vi "Xbox 2nd.vi"() -> (14 "Turn?":bool, 16 "Fire?":bool, 17 "Repelling Balls?":bool, 18 "Right Side?":bool, 19 "Collecting Balls?":bool, 20 "Viewer Select":T2(ring)=enum."Ball Camera", 21 "Hoop Select":T1(ring), 22 "Number Of Balls":i32, 23 "Shooting Manual Override?":bool, 24 "Ball Managment Manual Override?":bool, 25 "No Target Alert":bool, 26 "Manual Override Engaged?":bool, 27 "Aligning?":bool)   [LabVIEW 2011]
uses:
  Team Code/Robot Global Data.vi
panel:
  out "Current RPM":dbl
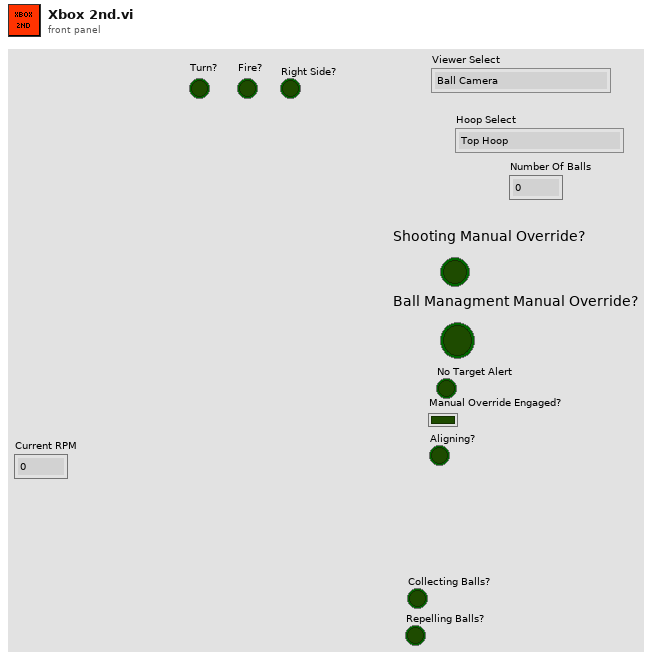
[diagram p1: front panel]
types:
  T1 = enum32{"Top Hoop", "Bottom Hoop", "Left Hoop", "Right Hoop"}
  T2 = enum32{"Target Camera", "Target Camera Mask", "Ball Camera", "Kinect Skeleton"}
  T3 = typedef "WPI_JoystickButtonState.ctl" = cluster{"Button 1":bool, "Button 2":bool, "Button 3":bool, "Button 4":bool, "Button 5":bool, "Button 6":bool, "Button 7":bool, "Button 8":bool, "Button 9":bool, "Button 10":bool, "Button 11":bool, "Button 12":bool}
  T4 = cluster{"Buttons":T3, "Axes":cluster{"axis 1 (x)":dbl, "axis 2 (y)":dbl, "axis 3 (throttle)":dbl, "axis 4":dbl, "axis 5":dbl, "axis 6":dbl}}
  T5 = cluster{"Position":cluster{"X Angle":dbl, "Raw Y":dbl, "Raw X":dbl}, "Distance (ft)":dbl, "BB Angle":dbl}
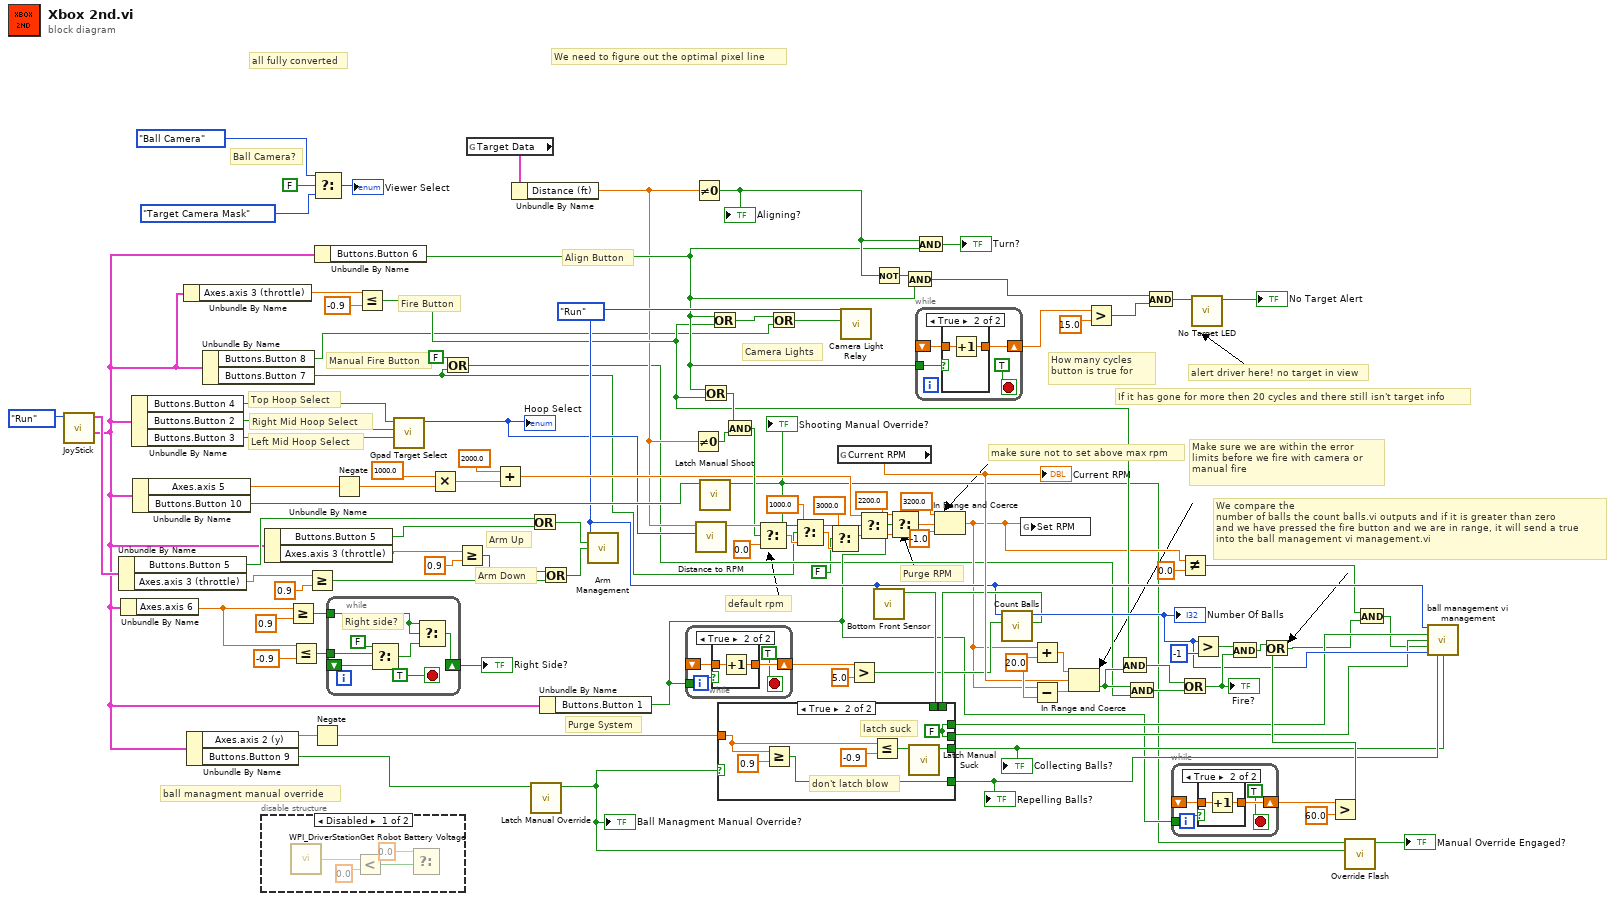
[diagram p0: block diagram]
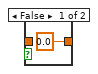
[diagram p2: hidden frame]
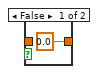
[diagram p4: hidden frame]
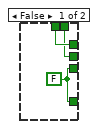
[diagram p5: hidden frame]
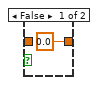
[diagram p6: hidden frame]
diagram:
  w96 = 20.0 ("y")
  w44 = enum16{"Init", "Run", "End"}."Run" ("Enum")
  # "all fully converted"
  # "default rpm"
  # "Make sure we are within the error limits before we fire with camera or manual fire"
  # "make sure not to set above max rpm"
  # "Purge System"
  # "Left Mid Hoop Select"
  # "Right Mid Hoop Select"
  # "Top Hoop Select"
  # "Purge RPM"
  # "We compare the \nnumber of balls the count balls.vi outputs and if it is greater than zero \nand we have pressed the fire button and we are in range, it will send a true\ninto the ball management vi management.vi"
  # "ball managment manual override"
  # "We need to figure out the optimal pixel line"
  # "Arm Down"
  # "Arm Up"
  # "Ball Camera?"
  # "Fire Button"
  # "Manual Fire Button"
  # "Camera Lights"
  # "Align Button"
  # "If it has gone for more then 20 cycles and there still isn't target info"
  # "How many cycles button is true for"
  # "alert driver here! no target in view"
  n1 = call "JoyStick.vi"("Enum"=enum16{"Init", "Run", "End"}."Run") -> ("JoyStick 3"=w34:T4, "JoyStick 1"=w43:T4)  [unwired: 7 in, 2 out]
  n2 = Unbundle By Name(w43) -> ("Buttons.Button 5"=w36:bool, "Axes.axis 3 (throttle)"=w30:dbl)
  n3 = Unbundle By Name(w34) -> ("Axes.axis 6"=w85:dbl)
  n4 = Unbundle By Name(w34) -> ("Buttons.Button 4"=w65:bool, "Buttons.Button 2"=w91:bool, "Buttons.Button 3"=w90:bool)
  n5 = Unbundle By Name(w34) -> ("Axes.axis 5"=w80:dbl, "Buttons.Button 10"=w60:bool)
  n6 = Unbundle By Name(w34) -> ("Axes.axis 3 (throttle)"=w32:dbl)
  n7 = Unbundle By Name(w34) -> ("Axes.axis 2 (y)"=w58:dbl, "Buttons.Button 9"=w59:bool)
  n8 = Unbundle By Name(w34) -> ("Buttons.Button 8"=w1:bool, "Buttons.Button 7"=w6:bool)
  n9 = disable-structure shown="Disabled" {
    frame Disabled {
      n10 = call <vilib>:"WPI_DriverStationGet Robot Battery Voltage.vi"() -> ("robot battery voltage"=w112:dbl)  [unwired: 14 in, 1 out]
      n11 = Less?(x=w112, y=0.0) -> (x < y?=w110:bool)
      n12 = Select(t=0.0, s=w110) -> ()  [unwired: 1 in, 1 out]
    }
    frame Enabled {
    }
  }
  n13 = Unbundle By Name(w34) -> ("Buttons.Button 5"=w37:bool, "Axes.axis 3 (throttle)"=w28:dbl)
  n14 = Greater Or Equal?(x=w85, y=0.9) -> (x >= y?=w83:bool)
  n15 = Less Or Equal?(x=w85, y=-0.9) -> (x <= y?=w82:bool)
  n16 = Greater Or Equal?(x=w30, y=0.9) -> (x >= y?=w29:bool)
  n17 = Negate(x=w58) -> (-x=w66:dbl)
  n18 = Select(t=T2."Ball Camera" ("Viewer Select"), s=FALSE, f=T2."Target Camera Mask" ("Viewer Select")) -> (s? t:f=→"Viewer Select":T2)
  n19 = Unbundle By Name(w34) -> ("Buttons.Button 6"=w40:bool)
  n20 = while {
    tunnel: w83 -> [w115]
    tunnel: w82 -> [w116]
    shift-right: [w117] -> w81
    shift-left: _ -> [w118]
    stop <- TRUE stop-if-true
    # "Right side?"
    n21 = Select(t=FALSE, s=w116, f=w118) -> (s? t:f=w119:bool)
    n22 = Select(t=w115, s=w115, f=w119) -> (s? t:f=w117:bool)
  }
  "Right Side?" <- w81
  n23 = Negate(x=w80) -> (-x=w67:dbl)
  n24 = Less Or Equal?(x=w32, y=-0.9) -> (x <= y?=w31:bool)
  n25 = call "Gpad Target Select.vi"("Left Hoop"=w90, "Right Hoop"=w91, "Top Hoop"=w65) -> ("Hoop Select"=w38:T1)  [unwired: 8 in]
  "Hoop Select" <- w38
  n26 = Multiply(x=1000.0, y=w67) -> (x*y=w78:dbl)
  n27 = Or(x=FALSE, y=w6) -> (x .or. y?=w11:bool)
  n28 = Greater Or Equal?(x=w28, y=0.9) -> (x >= y?=w27:bool)
  n29 = global read "Robot Global Data.vi" "Target Data"() -> (w56:T5)
  n30 = Add(x=2000.0, y=w78) -> (x+y=w76:dbl)
  n31 = Unbundle By Name(w56) -> ("Distance (ft)"=w19:dbl)
  n32 = Or(x=w36, y=w37) -> (x .or. y?=w42:bool)
  n33 = call "Latch Manual Override.vi"("Input"=w59) -> ("Latched"=w73:bool)  [unwired: 10 in]
  "Ball Managment Manual Override?" <- w73
  n34 = Unbundle By Name(w34) -> ("Buttons.Button 1"=w20:bool)
  n35 = Or(x=w27, y=w29) -> (x .or. y?=w41:bool)
  n36 = call "Arm Management.vi"("Enum"=w44, "Up Button"=w42, "Down Button"=w41) -> ()  [unwired: 13 in]
  n37 = while {
    tunnel: w20 -> [w123]
    shift-right: [w121] -> w23
    shift-left: _ -> [w122]
    stop <- TRUE stop-if-true
    n38 = case shown="True" w123 {
      tunnel: w122 -> [_ w126]
      tunnel: [0.0 w125] -> w121
      frame False {
      }
      frame True {
        n39 = Increment(x=w126) -> (x+1=w125:dbl)
      }
    }
  }
  n40 = Not Equal To 0?(x=w19) -> (x != 0?=w101:bool)
  n41 = Not Equal To 0?(x=w19) -> (x != 0?=w62:bool)
  "Aligning?" <- w62
  n42 = call "Distance to RPM.vi"("Distance"=w19, "Hoop"=w38) -> ("Shooter RPM"=w105:dbl)  [unwired: 8 in]
  n43 = call "Latch Manual Shoot.vi"("Input"=w60) -> ("Latched"=w10:bool)  [unwired: 10 in]
  "Shooting Manual Override?" <- w10
  n44 = Or(x=w40, y=w31) -> (x .or. y?=w39:bool)
  n45 = Or(x=w40, y=w31) -> (x .or. y?=w3:bool)
  n46 = And(x=w39, y=w101) -> (x .and. y?=w100:bool)
  n47 = Select(t=w105, s=w100, f=0.0) -> (s? t:f=w9:dbl)
  n48 = Or(x=w3, y=w1) -> (x .or. y?=w2:bool)
  n49 = Select(t=1000.0, s=w6, f=w9) -> (s? t:f=w8:dbl)
  n50 = Select(t=3000.0, s=FALSE, f=w8) -> (s? t:f=w12:dbl)
  n51 = global read "Robot Global Data.vi" "Current RPM"() -> (w46:dbl)
  "Current RPM" <- w46
  n52 = call "Camera Light Relay.vi"("Camera Light"=w2, "Enum"=w44) -> ()  [unwired: 10 in]
  n53 = Greater?(x=w23, y=5.0) -> (0:w21:bool)
  n54 = Select(t=w76, s=w10, f=w12) -> (s? t:f=w70:dbl)
  n55 = Not(x=w62) -> (.not. x?=w107:bool)
  n56 = call "Bottom Front Sensor.vi"("Enum"=w44) -> ("Bottom Front"=w52:bool)  [unwired: 10 in]
  n57 = Select(t=2200.0, s=w20, f=w70) -> (s? t:f=w69:dbl)
  n58 = And(x=w107, y=w40) -> (x .and. y?=w102:bool)
  n59 = And(x=w62, y=w40) -> (x .and. y?=→"Turn?":bool)
  n60 = while {
    tunnel: w40 -> [w130]
    shift-right: [w128] -> w103
    shift-left: _ -> [w129]
    stop <- TRUE stop-if-true
    n61 = case shown="True" w130 {
      tunnel: w129 -> [_ w133]
      tunnel: [0.0 w132] -> w128
      frame False {
      }
      frame True {
        n62 = Increment(x=w133) -> (x+1=w132:dbl)
      }
    }
  }
  n63 = In Range and Coerce(upper limit=3200.0, x=w69, lower limit=-1.0) -> (coerced(x)=w18:dbl)  [unwired: 1 out]
  n64 = call "Count Balls.vi"("Reset Ball Count?"=w21, "Mode"=w44) -> ("Bottom Back?"=w45:bool, "Number Of Balls"=w51:i32)  [unwired: 8 in]
  "Number Of Balls" <- w51
  n65 = case shown="True" w73 {
    tunnel: w66 -> [_ w141]
    tunnel: w52 -> [w135 _]
    tunnel: [w136 w140] -> w54
    tunnel: [w136 w139] -> w53
    tunnel: [w135 w137] -> w50
    tunnel: w45 -> [w134 _]
    tunnel: [w134 w137] -> w49
    frame False {
      w136 = FALSE
    }
    frame True {
      w137 = FALSE ("Run Conveyor Feeder?")
      # "latch suck"
      # "don't latch blow"
      n66 = Greater Or Equal?(x=w141, y=0.9) -> (x >= y?=w140:bool)
      n67 = Less Or Equal?(x=w141, y=-0.9 ("x")) -> (x <= y?=w138:bool)
      n68 = call "Latch Manual Suck.vi"("Input"=w138) -> ("Latched"=w139:bool)  [unwired: 10 in]
    }
  }
  "Collecting Balls?" <- w53
  "Repelling Balls?" <- w54
  n69 = global write "Robot Global Data.vi" "Set RPM"(w18) -> ()
  n70 = Add(x=w18, y=w96) -> (x+y=w95:dbl)
  n71 = Subtract(x=w18, y=w96) -> (x-y=w94:dbl)
  n72 = In Range and Coerce(upper limit=w95, x=w46, lower limit=w94) -> (In Range?=w93:bool)  [unwired: 1 out]
  n73 = Greater?(x=w103, y=15.0) -> (0:w61:bool)
  n74 = And(x=w31, y=w93) -> (x .and. y?=w98:bool)
  n75 = And(x=w93, y=w11) -> (x .and. y?=w97:bool)
  n76 = And(x=w102, y=w61) -> (x .and. y?=w35:bool)
  n77 = while {
    tunnel: w20 -> [w147]
    shift-right: [w145] -> w68
    shift-left: _ -> [w146]
    stop <- TRUE stop-if-true
    n78 = case shown="True" w147 {
      tunnel: w146 -> [_ w150]
      tunnel: [0.0 w149] -> w145
      frame False {
      }
      frame True {
        n79 = Increment(x=w150) -> (x+1=w149:dbl)
      }
    }
  }
  n80 = Not Equal?(x=w18, y=0.0) -> (x != y?=w15:bool)
  n81 = Or(x=w98, y=w97) -> (x .or. y?=w89:bool)
  "Fire?" <- w89
  n82 = call "No Target LED.vi"("Thing 1"=w35) -> ("Flashy the LED"=→"No Target Alert":bool)  [unwired: 10 in]
  n83 = Greater?(x=w51, y=-1) -> (0:w87:bool)
  n84 = And(x=w87, y=w89) -> (x .and. y?=w75:bool)
  n85 = Greater?(x=w68, y=60.0) -> (0:w55:bool)
  n86 = Or(x=w75, y=w55) -> (x .or. y?=w16:bool)
  n87 = call "Override Flash.vi"("Thing 2"=w73, "Thing 1"=w10) -> ("Flashy the LED"=→"Manual Override Engaged?":bool)  [unwired: 9 in]
  n88 = And(x=w15, y=w16) -> (x .and. y?=w14:bool)
  n89 = call "ball management vi management.vi"("Enum"=w44, "Bottom Front Sensor"=w50, "Bottom Back Sensor"=w49, "Shoot?"=w14, "# of Balls"=w51, "Manual Blow Hard?"=w54, "Manual SUCK-IT HARD!!!!"=w53) -> ()  [unwired: 9 in]
